vi "FTS Setup Virtual Source_RS.vi"(8 "error in (no error)":errorcluster, 10 "source type RS (LLD/DFB 1530nm)":T1=enum."VIRTUAL_REDSTONE_SOURCE_LLD_DFB_1530", 11 "specIndex":u16) -> (0 "error out":errorcluster, 3 "function return":i32)   [LabVIEW 2010, in "FTSLib.lvlib"]
doc: "int __cdecl FTS_SetupVirtualSource(unsigned short specIndex, VIRTUAL_SOURCE_TYPE type, virtual_source_parameter_t *parameters);"
uses:
  FTSLib.lvlib
  _misc/Thorlabs_FTS_misc.llb/OSA_virtualSource_RS.ctl
  FTSLib.dll
  OSA20X_misc.lvlib
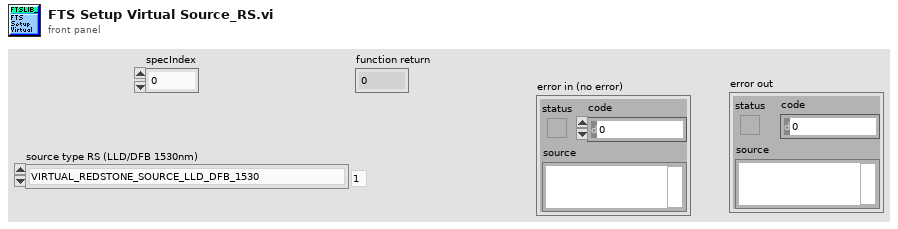
[diagram p1: front panel]
types:
  T1 = typedef "OSA20X_misc.lvlib/OSA_virtualSource_RS.ctl" = enum16{"VIRTUAL_REDSTONE_SOURCE_UNKNOWN", "VIRTUAL_REDSTONE_SOURCE_LLD_DFB_1530", "VIRTUAL_REDSTONE_SOURCE_SLD_1550nm", "VIRTUAL_REDSTONE_SOURCE_LASER_4600nm", "VIRTUAL_REDSTONE_SOURCE_BLACKBODY1500K", "VIRTUAL_REDSTONE_SOURCE_BLACKBODY1500K_H2O"}
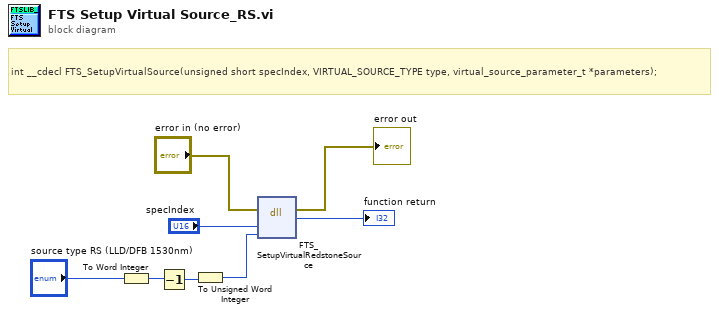
[diagram p0: block diagram]
diagram:
  # "int __cdecl FTS_SetupVirtualSource(unsigned short specIndex, VIRTUAL_SOURCE_TYPE type, virtual_source_parameter_t *parameters);"
  n1 = To Word Integer(number="source type RS (LLD/DFB 1530nm)") -> (16bit integer=w4:i16)
  n2 = Decrement(x=w4) -> (x-1=w3:i16)
  n3 = To Unsigned Word Integer(number=w3) -> (unsigned 16bit integer=w2:u16)
  n4 = dll-call lib="FTSLib.*" fn="FTS_SetupVirtualRedstoneSource"(error in="error in (no error)", "specIndex"="specIndex", "sourceType"=w2) -> (error out=→"error out":errorcluster, "return type"=→"function return":i32)  [unwired: 4 in, 1 out]
